vi "Inverse Complex FFT.vi"(10 "shift?":bool, 11 "FFT {X}":cdb[](array[numeric])) -> (0 "error":i32, 3 "X":cdb[](array[numeric]))   [LabVIEW 2010, in "NI_AALPro.lvlib"]
doc: "Computes the inverse discrete Fourier transform (IDFT) of the input sequence <B>FFT {X}</B>. You must manually select the polymorphic instance you want to use."
uses:
  NI_AALPro.lvlib
  lvanlys.dll
panel:
  # "Inverse Complex FFT"
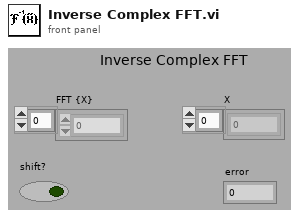
[diagram p1: front panel]
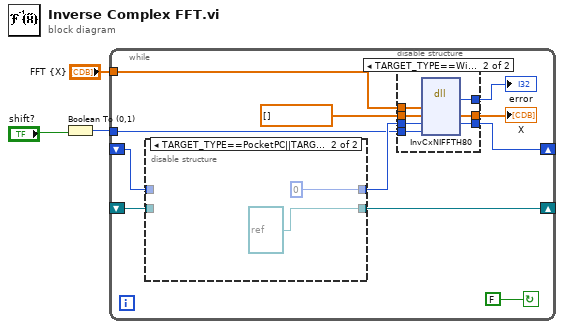
[diagram p0: block diagram]
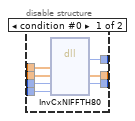
[diagram p2: hidden frame]
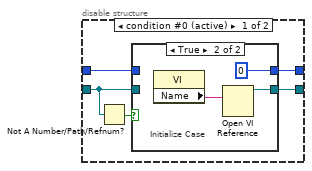
[diagram p3: hidden frame]
diagram:
  n1 = Boolean To (0,1)(Boolean="shift?") -> (0, 1=w1:i16)
  n2 = while {
    shift-left: _ -> [w10]
    shift-right: [w11] -> _
    tunnel: "FFT {X}" -> [w14]
    shift-right: [w7] -> _
    shift-left: _ -> [w8]
    tunnel: w1 -> [w6]
    stop <- FALSE continue-if-true
    n3 = disable-structure shown="TARGET_TYPE==PocketPC||TARGET_TYPE==PalmOS||TARGET_TYPE==FPGA||TARGET_TYPE==Embedded" {
      disable-tunnel: w8 -> [w31 _]
      disable-tunnel: [w32 refnum<vi> refnum ("VI Refnum")] -> w7
      disable-tunnel: w10 -> [w30 _]
      disable-tunnel: [w29 0 ("t")] -> w9
      frame condition #0 (active) {
        n4 = Not A Number/Path/Refnum?(number/path/refnum=w31) -> (NaN/Path/Refnum?=w33:bool)
        n5 = case shown="True" w33 {
          tunnel: [w35 w37] -> w32
          tunnel: w31 -> [w35 _]
          tunnel: w30 -> [w34 _]
          tunnel: [w34 0 ("error")] -> w29
          frame False {
          }
          frame True {
            # "Initialize Case"
            n6 = property class="VI"() -> ("Name"=w36:string)  [unwired: 2 in, 2 out]
            n7 = Open VI Reference(vi path=w36) -> (vi reference=w37:refnum<vi>)  [unwired: 5 in, 1 out]
          }
        }
      }
      frame condition #1 {
      }
    }
    n8 = disable-structure shown="TARGET_TYPE==Windows||TARGET_TYPE==Mac||TARGET_TYPE==Unix" {
      disable-tunnel: w14 -> [w21 w28]
      disable-tunnel: [w20 w27] -> w13
      disable-tunnel: [w19 w26] -> w5
      disable-tunnel: [w18 w25] -> w11
      disable-tunnel: w9 -> [w17 w24]
      disable-tunnel: w6 -> [w16 w23]
      disable-tunnel: cdb[] [] ("X") -> [w15 w22]
      frame condition #0 {
        n9 = dll-call lib="C:/Program Files/National Instruments/LabVIEW 2010/resource/lvanlys.dll" fn="InvCxNIFFTH80"("FFT {X}"=w21, w15, "tbl"=w17, "shift"=w16) -> (w20:i32, w19:cdb[], "tbl"=w18:i32)  [unwired: 5 in, 2 out]
      }
      frame condition #1 (active) {
        n10 = dll-call lib="C:/Program Files/National Instruments/LabVIEW 2010/resource/lvanlys.dll" fn="InvCxNIFFTH80"("xH"=w28, "yH"=w22, "tbl"=w24, "shift"=w23) -> ("return type"=w27:i32, "yH"=w26:cdb[], "tbl"=w25:i64)  [unwired: 5 in, 2 out]
      }
    }
    "X" <- w5
    "error" <- w13
  }
